vi "ReadPointFromMem.vi"(11 "PointNum":u32) -> (3 "Point":cluster{"X":i32, "Y":i32, "Z":i32})   [LabVIEW 2014]
uses:
  <vilib>/Platform/TimedLoop/XDataNode/timing_clust.ctl
  <vilib>/Platform/TimedLoop/XDataNode/nitl_modes.ctl
  <vilib>/Platform/TimedLoop/XDataNode/wakeup.ctl
  <vilib>/rvi/Emulation/niFpgaSctlEmulationGetInTimedLoop.vi
  <vilib>/rvi/Emulation/niFpgaEmulationReportErrorSimple.vi
  <vilib>/rvi/Emulation/niFpgaGetClockAttributes.vi
  <vilib>/rvi/Emulation/niFpgaCriticalErrorInLSC.vi
  <vilib>/rvi/eio/common/nirviEmuTemplateMethod_errors.vi
  <vilib>/Platform/TimedLoop/XDataNode/XDataNode.xnode
  <vilib>/eio/EIONode/EIONode.xnode
  <vilib>/Platform/TimedLoop/XDataNode/XDNodeRunTimeDep.lvlib
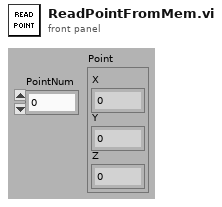
[diagram p1: front panel]
types:
  T1 = typedef "XDNodeRunTimeDep.lvlib/timing_clust.ctl" = cluster{"Expected End [f-1]":u64, "Actual End [f-1]":u64, "Finished Late? [f-1]":bool, "Expected End [i-1]":u64, "Actual End [i-1]":u64, "Finished Late? [i-1]":bool, "Expected Start [i]":u64, "Actual Start [i]":u64, "Expected Start [f]":u64, "Actual Start [f]":u64, "Source Name":string, "Structure Name":string, "Period":i64, "Deadline":i64, "Offset":i64, "Start":i64, "Priority":i32, "Timeout":i32, "Mode":T2, "Wakeup Reason":T3, "Error":errorcluster, "Source Type":string, "Secondary Source Type":string, "Global End Time":u64, "Global Start Time":u64, "Frame Duration":u64, "Iteration Duration":u64, "Assigned CPU":i32, "I/O Scan Engine Mode":u32}
  T2 = typedef "XDNodeRunTimeDep.lvlib/nitl_modes.ctl" = enum32{"No Change", "Process missed periods, maintain original phase", "Discard missed periods, maintain original phase", "Process missed periods, ignore original phase", "Discard missed periods, ignore original phase"}
  T3 = typedef "XDNodeRunTimeDep.lvlib/wakeup.ctl" = enum32{"Normal", "Aborted", "Asynchronous wakeup", "Timing source error", "Timed loop error", "Timeout"}
  T4 = enum16{"ReadXY", "XYstrobe", "ReadZ", "ZStrobe", "Done"}
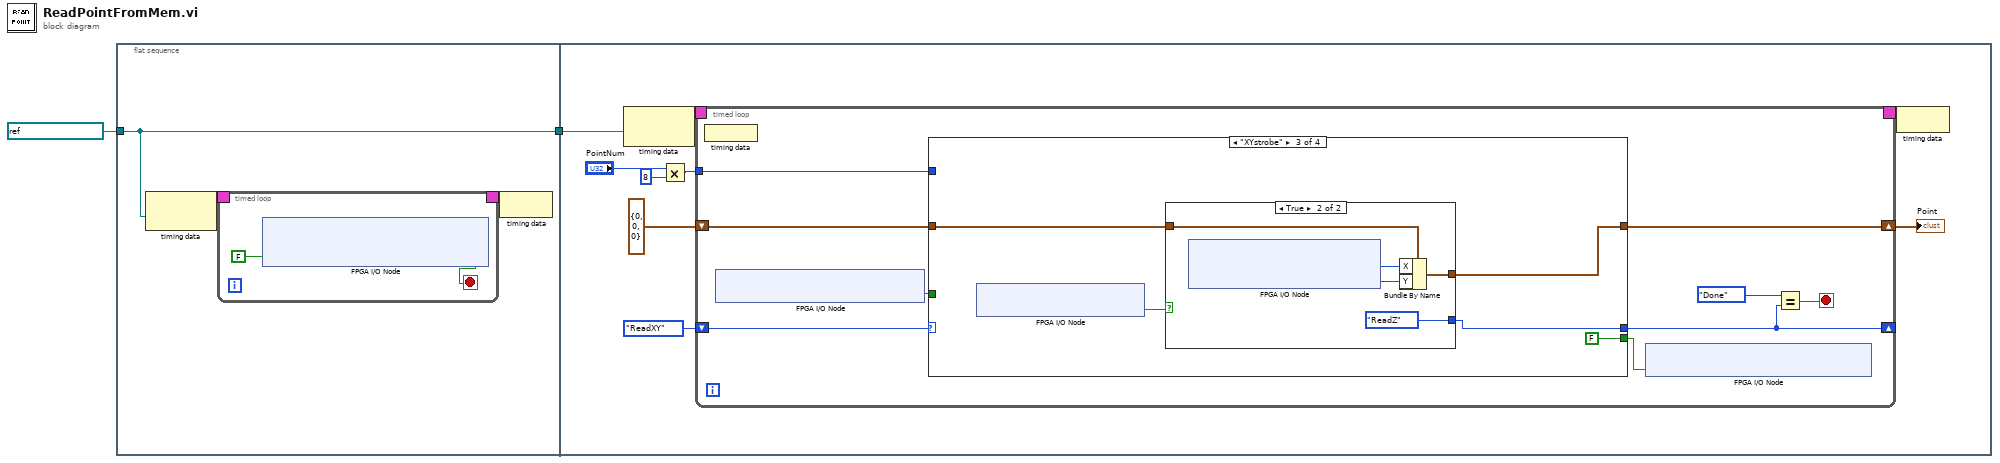
[diagram p0: block diagram]
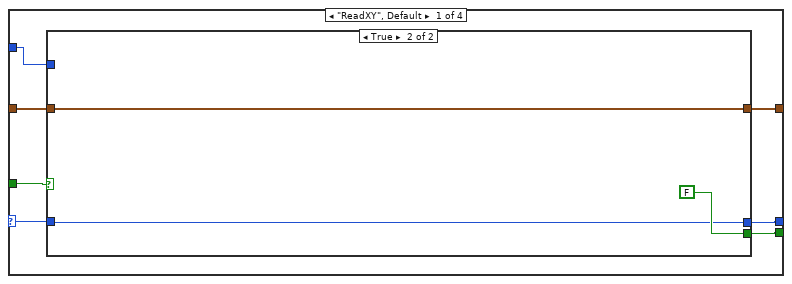
[diagram p2: hidden frame]
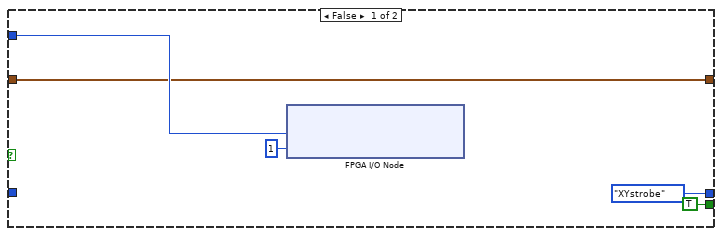
[diagram p3: hidden frame]
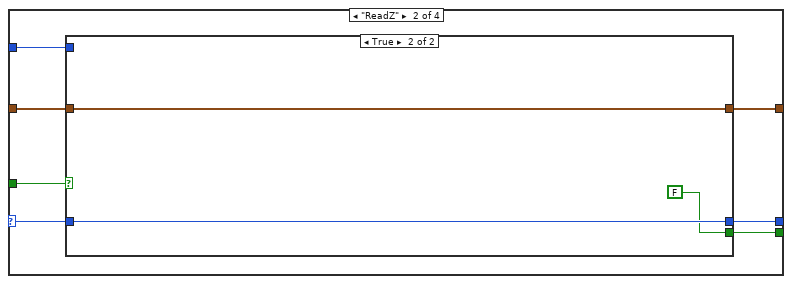
[diagram p4: hidden frame]
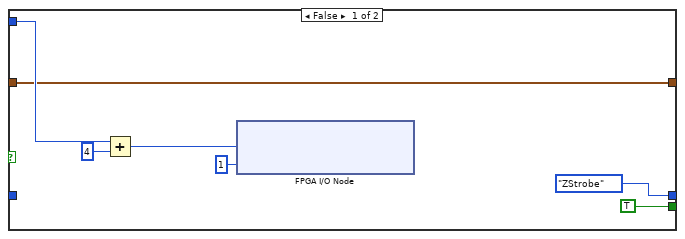
[diagram p5: hidden frame]
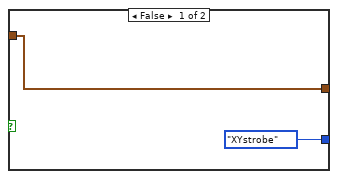
[diagram p6: hidden frame]
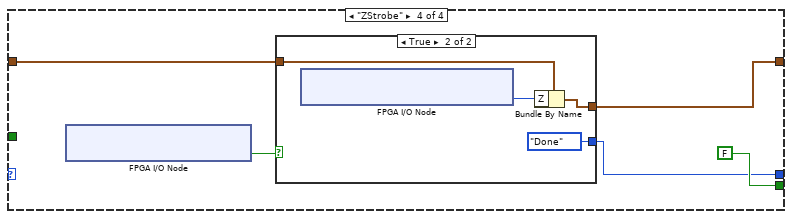
[diagram p7: hidden frame]
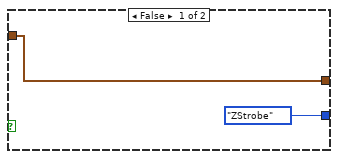
[diagram p8: hidden frame]
diagram:
  n1 = flat-sequence {
    tunnel: refnum<k21> "100 MHz Clock" ("Source Name") -> [w3]
    tunnel: [w3] -> w1
    tunnel: w1 -> [w14]
    frame #0 {
      n2 = node-c288(w3) -> (w5:T1)
      n3 = timed-loop {
        timing: w5 -> [_]
        timing-out: [_] -> w4
        stop <- w7 stop-if-true
        n4 = xnode "FPGA I/O Node"("DRAM Bank 0\\Command_Write_Enable"=FALSE ("DRAM Bank 0\\Command_Write_Enable")) -> ("DRAM Bank 0\\Initialization_Done"=w7:bool)  [unwired: 2 in, 2 out]
      }
      n5 = node-c288(w4) -> ()
    }
    frame #1 {
      n6 = node-c288(w14) -> (w22:T1)
      n7 = Multiply(x="PointNum", y=i16 8) -> (x*y=w18:u32)
      n8 = timed-loop {
        timing: w22 -> [_]
        timing-out: [_] -> w21
        tunnel: w18 -> [w29]
        shift-right: [w25] -> _
        shift-left: T4."ReadXY" -> [w30]
        shift-right: [w27] -> w15
        shift-left: cluster{"X":i32, "Y":i32, "Z":i32} {"X"=0, "Y"=0, "Z"=0} ("Point") -> [w28]
        stop <- w26 stop-if-true
        n9 = node-c288() -> ()  [unwired: 1 in]
        n10 = xnode "FPGA I/O Node"() -> ("DRAM Bank 0\\Command_FIFO_Full"=w23:bool)  [unwired: 1 in, 1 out]
        n11 = case shown="\"XYstrobe\"" w30 {
          selector: w30 -> [w34 w47 _ _]
          tunnel: [w37 w51 w64 w76] -> w25
          tunnel: [w36 w52 FALSE FALSE] -> w31
          tunnel: w29 -> [w38 w53 _ _]
          tunnel: w28 -> [w33 w49 w66 w79]
          tunnel: [w32 w48 w65 w77] -> w27
          tunnel: w23 -> [w35 w50 _ _]
          frame "ReadXY", Default {
            n12 = case shown="True" w35 {
              tunnel: w38 -> [w43 _]
              tunnel: [enum16{"ReadXY", "XYstrobe", "ReadZ", "ZStrobe"}."XYstrobe" w45] -> w37
              tunnel: [TRUE FALSE] -> w36
              tunnel: w34 -> [_ w45]
              tunnel: w33 -> [w39 w44]
              tunnel: [w39 w44] -> w32
              frame False {
                n13 = xnode "FPGA I/O Node"("DRAM Bank 0\\Address"=w43, "DRAM Bank 0\\Command"=u8 1 ("DRAM Bank 0\\Command")) -> ()  [unwired: 2 in, 2 out]
              }
              frame True {
              }
            }
          }
          frame "ReadZ" {
            n14 = case shown="True" w50 {
              tunnel: w53 -> [w59 _]
              tunnel: [TRUE FALSE] -> w52
              tunnel: [enum16{"ReadXY", "XYstrobe", "ReadZ", "ZStrobe"}."ZStrobe" w62] -> w51
              tunnel: w49 -> [w54 w63]
              tunnel: [w54 w63] -> w48
              tunnel: w47 -> [_ w62]
              frame False {
                n15 = Add(x=w59, y=u32 4) -> (x+y=w57:u32)
                n16 = xnode "FPGA I/O Node"("DRAM Bank 0\\Address"=w57, "DRAM Bank 0\\Command"=u8 1 ("DRAM Bank 0\\Command")) -> ()  [unwired: 2 in, 2 out]
              }
              frame True {
              }
            }
          }
          frame "XYstrobe" {
            n17 = xnode "FPGA I/O Node"() -> ("DRAM Bank 0\\Read_Strobe"=w67:bool)  [unwired: 1 in, 1 out]
            n18 = case shown="True" w67 {
              tunnel: w66 -> [w70 w75]
              tunnel: [w70 w72] -> w65
              tunnel: [enum16{"ReadXY", "XYstrobe", "ReadZ", "ZStrobe"}."XYstrobe" enum16{"ReadXY", "XYstrobe", "ReadZ", "ZStrobe"}."ReadZ"] -> w64
              frame False {
              }
              frame True {
                n19 = xnode "FPGA I/O Node"() -> ("DRAM Bank 0\\Read_Data_Upper"=w74:u64, "DRAM Bank 0\\Read_Data_Lower"=w73:u64)  [unwired: 2 in, 2 out]
                n20 = Bundle By Name(cluster=w75, "X"=w74, "Y"=w73) -> (w72:cluster{"X":i32, "Y":i32, "Z":i32})
              }
            }
          }
          frame "ZStrobe" {
            n21 = xnode "FPGA I/O Node"() -> ("DRAM Bank 0\\Read_Strobe"=w80:bool)  [unwired: 1 in, 1 out]
            n22 = case shown="True" w80 {
              tunnel: w79 -> [w82 w86]
              tunnel: [w82 w84] -> w77
              tunnel: [enum16{"ReadXY", "XYstrobe", "ReadZ", "ZStrobe"}."ZStrobe" T4."Done"] -> w76
              frame False {
              }
              frame True {
                n23 = xnode "FPGA I/O Node"() -> ("DRAM Bank 0\\Read_Data_Upper"=w85:u64)  [unwired: 1 in, 1 out]
                n24 = Bundle By Name(cluster=w86, "Z"=w85) -> (w84:cluster{"X":i32, "Y":i32, "Z":i32})
              }
            }
          }
        }
        n25 = xnode "FPGA I/O Node"("DRAM Bank 0\\Command_Write_Enable"=w31) -> ()  [unwired: 1 in, 1 out]
        n26 = Equal?(x=T4."Done", y=w25) -> (x = y?=w26:bool)
      }
      "Point" <- w15
      n27 = node-c288(w21) -> ()
    }
  }
